vi "get channels test.vi"() -> (0 "error out":errorcluster, 3 "channels match":bool)   [LabVIEW 2015, in "E2E Tag Exchange tests.lvlib"]
doc: "Tests the 'Get Channels' VI of the Configuration class."
uses:
  E2E Tag Exchange tests.lvlib
  module/configuration/E2E Tag Exchange configuration.lvclass
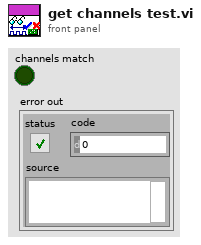
[diagram p1: front panel]
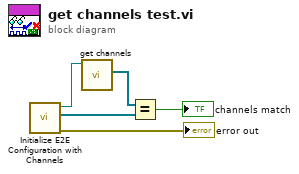
[diagram p0: block diagram]
diagram:
  n1 = call "Initialize E2E Configuration with Channels.vi"() -> ("error out"=→"error out":errorcluster, "Random Channels Added"=w2:refnum<class "TBM channel.lvclass">[], "Initialized E2E configuration"=w1:refnum<class "E2E Tag Exchange configuration.lvclass">)  [unwired: 9 in]
  n2 = call-dynamic "get channels.vi"("E2E configuration in"=w1) -> ("channels"=w5:refnum<class "TBM channel.lvclass">[])  [unwired: 9 in, 1 out]
  n3 = Equal?(x=w5, y=w2) -> (x = y?=→"channels match":bool)
